vi "ReadPropBand.vi"() -> ()   [LabVIEW 2013, in "ovenCtrl.lvlib"]
uses:
  ovenCtrl.lvlib
panel:
  out "Prop. Band":dbl format="%.2f"
  in  "error in (no error)":errorcluster
  out "error out":errorcluster
  in  "Port Number":u16=2000
  in  "IP Address":string="192.168.12.200"
  # "Inputs"
  # "Outputs"
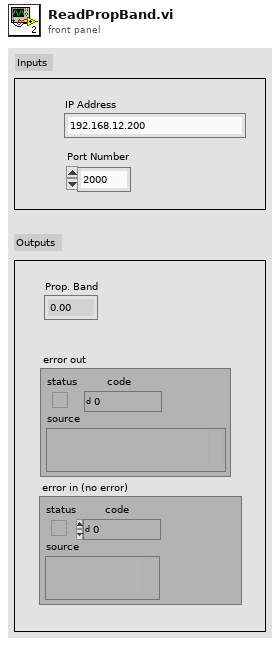
[diagram p1: front panel]
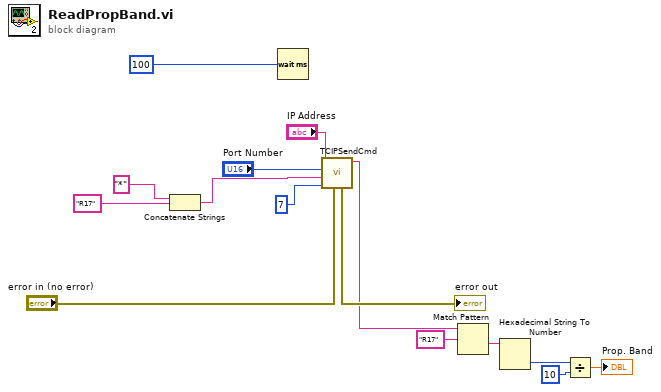
[diagram p0: block diagram]
diagram:
  n1 = Concatenate Strings("*" ("string"), "R17" ("string")) -> (w10:string)
  n2 = Wait (ms)(milliseconds to wait=u32 100) -> ()  [unwired: 1 out]
  n3 = call "TCIPSendCmd.vi"("error in (no error)"="error in (no error)", "bytes to read"=7, "Command"=w10, "Port Number"="Port Number", "IP Address"="IP Address") -> ("Output Reading"=w3:string, "error out"=→"error out":errorcluster)  [unwired: 5 in]
  n4 = Match Pattern(string=w3, regular expression="R17") -> (after substring=w1:string)  [unwired: 1 in, 3 out]
  n5 = Hexadecimal String To Number(string=w1) -> (number=w5:u32)  [unwired: 2 in, 1 out]
  n6 = Divide(x=w5, y=u32 10) -> (x/y=→"Prop. Band":dbl)
